vi "MccHat_Test.vi"() -> ()   [LabVIEW 2019]
panel:
  in  "interval":u32=1000
  out "readings":cluster{i32, i32, dbl}[](array[cluster])
  out "status_init":bool
  out "status_read":bool
  out "N":i32
  in  "stop":bool
  in  "port":u16=7020
  in  "address":string="10.0.0.21"
  out "error out":errorcluster
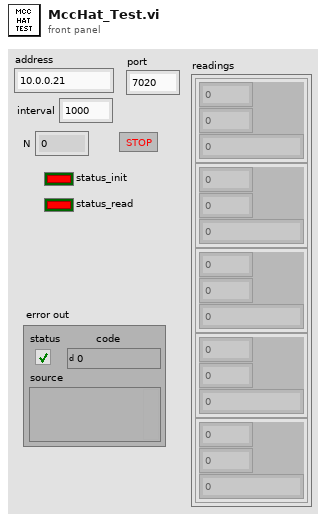
[diagram p1: front panel]
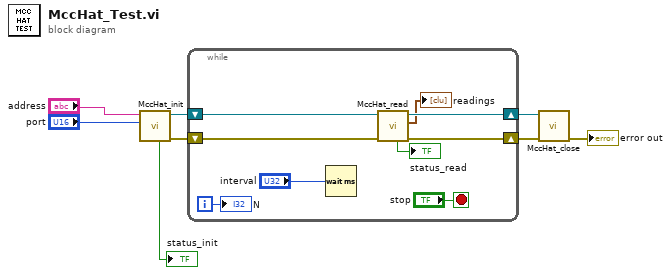
[diagram p0: block diagram]
diagram:
  n1 = call "MccHat_init.vi"("port"="port", "address"="address") -> ("error out"=w5:errorcluster, "conn_id"=w6:refnum<k5>, "status"=→"status_init":bool)  [unwired: 7 in]
  n2 = while {
    shift-right: [w12] -> w2
    shift-left: w6 -> [w15]
    shift-right: [w11] -> w4
    shift-left: w5 -> [w14]
    i -> [w13]
    stop <- "stop" stop-if-true
    n3 = Wait (ms)(milliseconds to wait="interval") -> ()  [unwired: 1 out]
    n4 = call "MccHat_read.vi"("error in"=w14, "conn_id_in"=w15) -> ("error out"=w11:errorcluster, "readings"=→"readings":cluster{i32, i32, dbl}[], "conn_id_out"=w12:refnum<k5>, "status"=→"status_read":bool)  [unwired: 6 in]
    "N" <- w13
  }
  n5 = call "MccHat_close.vi"("error in"=w4, "conn_id"=w2) -> ("error out"=→"error out":errorcluster)  [unwired: 8 in, 1 out]
